vi "Frame Editor.vi"(8 "error in":errorcluster, 11 "Input File":path) -> (0 "error out":errorcluster, 1 "Cancelled":bool, 2 "Output Map":T3 {"value"."Type of Frame" items=["Raw Frame", "UDP/IP Tx Gen", "Tx UDP"]; "value"."Data" format="%.0x"}, 3 "Currently Loaded file":path)   [LabVIEW 2020, in "FrameEditor.lvlib"]
doc: "This template is for the Queued Message Handler design pattern.\n\nThe Event Handling Loop generates messages based on user interface actions.\n\nThe Message Handling Loop processes messages generated by the Event Handling Loop, or by other messages. The messages are string values, so new messages can be added easily to the Message Cases case structure in the Message Handling Loop. Each message cluster can also provide an optional value for Message Data, which is a variant that can be converted to whatever message-specific data is required."
uses:
  FrameEditor.lvlib
  controls/Type of Payload.ctl
  controls/Payload Map.ctl
  controls/Payload Record Type.ctl
  controls/UI Data.ctl
  <instrlib>/AIM GmbH/_AIM 664/helpers/EthFrameManagement/controls/arinc664_mac_src_info.ctl
  <instrlib>/AIM GmbH/_AIM 664/helpers/EthFrameManagement/controls/arinc664_ip_src_info.ctl
  support/Message Queue/Enqueue Message (Single).vi
  <instrlib>/AIM GmbH/_AIM 664/helpers/EthFrameManagement/Create Payload (Constant).vi
  <instrlib>/AIM GmbH/_AIM 664/helpers/EthFrameManagement/Create Payload (Increment).vi
  <instrlib>/AIM GmbH/_AIM 664/helpers/EthFrameManagement/Create Payload (Random).vi
  <vilib>/Utility/error.llb/Error Cluster From Error Code.vi
  <vilib>/ErrorRing/Error Ring.xnode
  support/Message Queue/Message Queue.lvlib
  support/User Event - Stop/User Event - Stop.lvlib
  <instrlib>/AIM GmbH/_AIM 664/AIM664LV.lvlib
  <instrlib>/AIM GmbH/_AIM 664/helpers/EthFrameManagement/EthFrameManagement.lvlib
panel:
  in  "Payloads":string(tree)
  in  "Header Information":T1={"Inter Frame Gap"=0, "Packet Group Wait Time"=10000, "Payload Buffer Mode"=0, "Payload Generation Mode"=0, "Preamble Count"=7, "Skew"=0, "Net Select"=4, "Frame Start Mode"=1, "Physical Error Injection"=0, "Sequence Number Init"=65535, "Sequence Number Offset"=65535} {"Net Select" items=["FDX_TX_FRAME_DLY_A"=0, "FDX_TX_FRAME_DLY_B"=1, "FDX_TX_FRAME_BOTH "=3, "FDX_TX_FRAME_ONLY_A"=4, "FDX_TX_FRAME_ONLY_B "=5]; "Frame Start Mode" items=["FDX_TX_FRAME_START_IFG", "FDX_TX_FRAME_START_PGWT", "FDX_TX_FRAME_START_TRG"]; "Physical Error Injection" items=["FDX_TX_FRAME_ERR_OFF"=0, "FDX_TX_FRAME_ERR_CRC"=1, "FDX_TX_FRAME_ERR_ALI"=2, "FDX_TX_FRAME_ERR_PRE"=4, "FDX_TX_FRAME_ERR_PHY"=8]; "Sequence Number Init" items=["FDX_TX_FRAME_SEQ_INIT_AUTO"=65535]; "Sequence Number Offset" items=["FDX_TX_FRAME_SEQ_OFFS_AUTO "=65535]; "Payload Generation Mode" items=["FDX_TX_FRAME_PGM_USER"=0, "FDX_TX_FRAME_PGM_IP_PART"=1, "FDX_TX_FRAME_PGM_IP_FULL"=2, "FDX_TX_FRAME_PGM_IP_PART_TT"=10, "FDX_TX_FRAME_PGM_IP_FULL_TT"=20]; "Payload Buffer Mode" items=["FDX_TX_FRAME_PBM_STD", "FDX_TX_FRAME_PBM_MAC", "FDX_TX_FRAME_PBM_UDP"]}
  in  "Type of Frame":T2=1 items=["Raw Frame", "UDP/IP Tx Gen", "Tx UDP"]
  out "option":u32
  in  "Payload ID":string
  in  "Tab Control":enum32{"Raw ", "Page 1", "Page 2"}(tab)
  out "Frame Size":u32=17
  in  "Headers":u8[](array[numeric])=[0, 0, 0, 0, 0, 0, 0, 0, 0, 0, 0, 0, 0, 0, 0, 0, 0] format="%02x"
  in  "UDP Source Port":u16=1
  in  "UDP Destination Port":u16=1
  in  "VL Id":u16=60
  in  "Domain ID":u8=1
  in  "Side ID":u8=1
  in  "Location ID":u8=1
  in  "Interface ID":u8=1
  in  "Partition ID":u8=1
  out "Source IP":string
  out "Destination MAC":string
  out "Source MAC":string
  out "Destination IP":string
  out "Frame Data":string[][](table)
  in  "Increment":u8=1 format="%.0x"
  in  "Start":u8=65 format="%02x"
  in  "Fill Value":u8=10 format="%02x"
  in  "Random Payload":bool
  in  "Increment Payload":bool
  in  "Fill Payload":bool
  in  "Bit Length":u16(ring) items=["Byte (8 bits)", "Word (16 bits)", "Long (32 bits)", "Quad (64 bits)"]
  in  "Clear Payload":bool
  in  "Payload Size":u32=17
  in  "Payload":u8[](array[numeric])=[0, 0, 0, 0, 0, 0, 0, 0, 0, 0, 0, 0, 0, 0, 0, 0, 0] format="%02x"
  in  "Cancel":bool
  in  "Load":bool
  in  "Save":bool
  in  "Remove":bool
  in  "Add / Update":bool
  in  "Exit":bool
  out "Display Message":string
  # "0-13 index: MAC Header\n14-34 index: IP Header\n35-43 index: UDP Header"
  # "Auto-generate Payload"
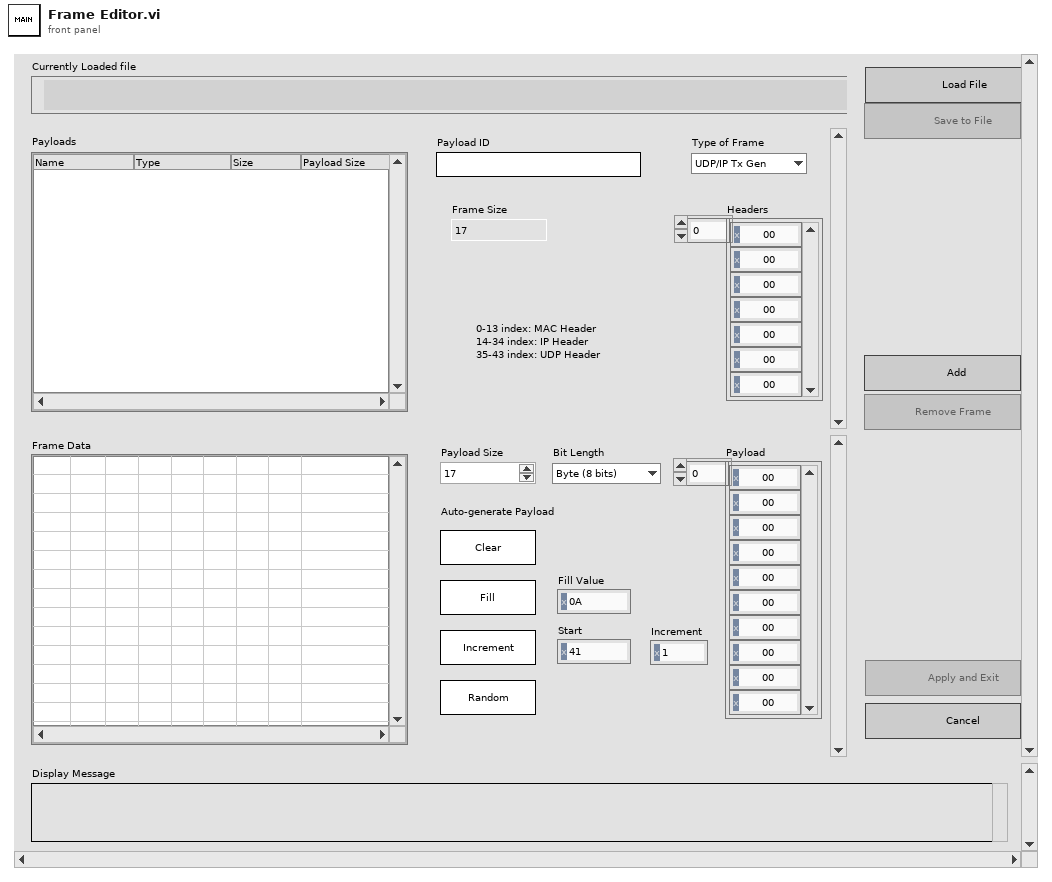
[diagram p1: front panel]
types:
  T1 = cluster{"Inter Frame Gap":u32, "Packet Group Wait Time":u32, "Payload Buffer Mode":u8, "Payload Generation Mode":u8, "Preamble Count":u8, "Skew":u32, "Net Select":u8, "Frame Start Mode":u8, "Physical Error Injection":u32, "Sequence Number Init":u16, "Sequence Number Offset":u16}
  T2 = typedef "Type of Payload.ctl" = u16
  T3 = typedef "Payload Map.ctl" = map{string, T4}
  T4 = typedef "Payload Record Type.ctl" = cluster{"Data":u8[], "Type of Frame":T2}
  T5 = typedef "UI Data.ctl" = cluster{"changesPending":bool, "String <Replace Me>":string, "Numeric <Replace Me>":dbl, "Add":refnum<vi>, "Remove":refnum<vi>, "Data Display Ref":refnum<vi>, "Exit Button Ref":refnum<vi>, "Load":refnum<vi>, "Save":refnum<vi>, "Payload ID":refnum<vi>, "Type of Frame":refnum<vi>}
  T6 = typedef "FrameEditor.lvlib/Message Queue.lvlib/All Message Queues.ctl" = cluster{"UI":refnum<queue>}
  T7 = cluster{"Left Cell String":string, "Child Text":string[], "Child Tag":string, "Item Indent":i32, "Child Only?":bool, "Glyph Index":i32}[]
  T8 = enum8{"Enabled", "Disabled", "Disabled and Grayed Out"}
  T9 = enum16{"open", "replace", "create", "open or create", "replace or create", "replace or create with confirmation"}
  T10 = typedef "EthFrameManagement.lvlib/arinc664_ip_src_info.ctl" = cluster{"domainID":u8, "sideID":u8, "locationID":u8, "partitionID":u8}
  T11 = typedef "EthFrameManagement.lvlib/arinc664_mac_src_info.ctl" = cluster{"domainID":u8, "sideID":u8, "locationID":u8, "interfaceID":u8}
  T12 = cluster{"Domain ID":u8, "Side ID":u8, "Location ID":u8, "Interface ID":u8, "Partition ID":u8}
  T13 = typedef "AIM664LV.lvlib/queue_data_full.ctl" = cluster{"domainID":u8, "sideID":u8, "locationID":u8, "interfaceID":u8, "partitionID":u8}
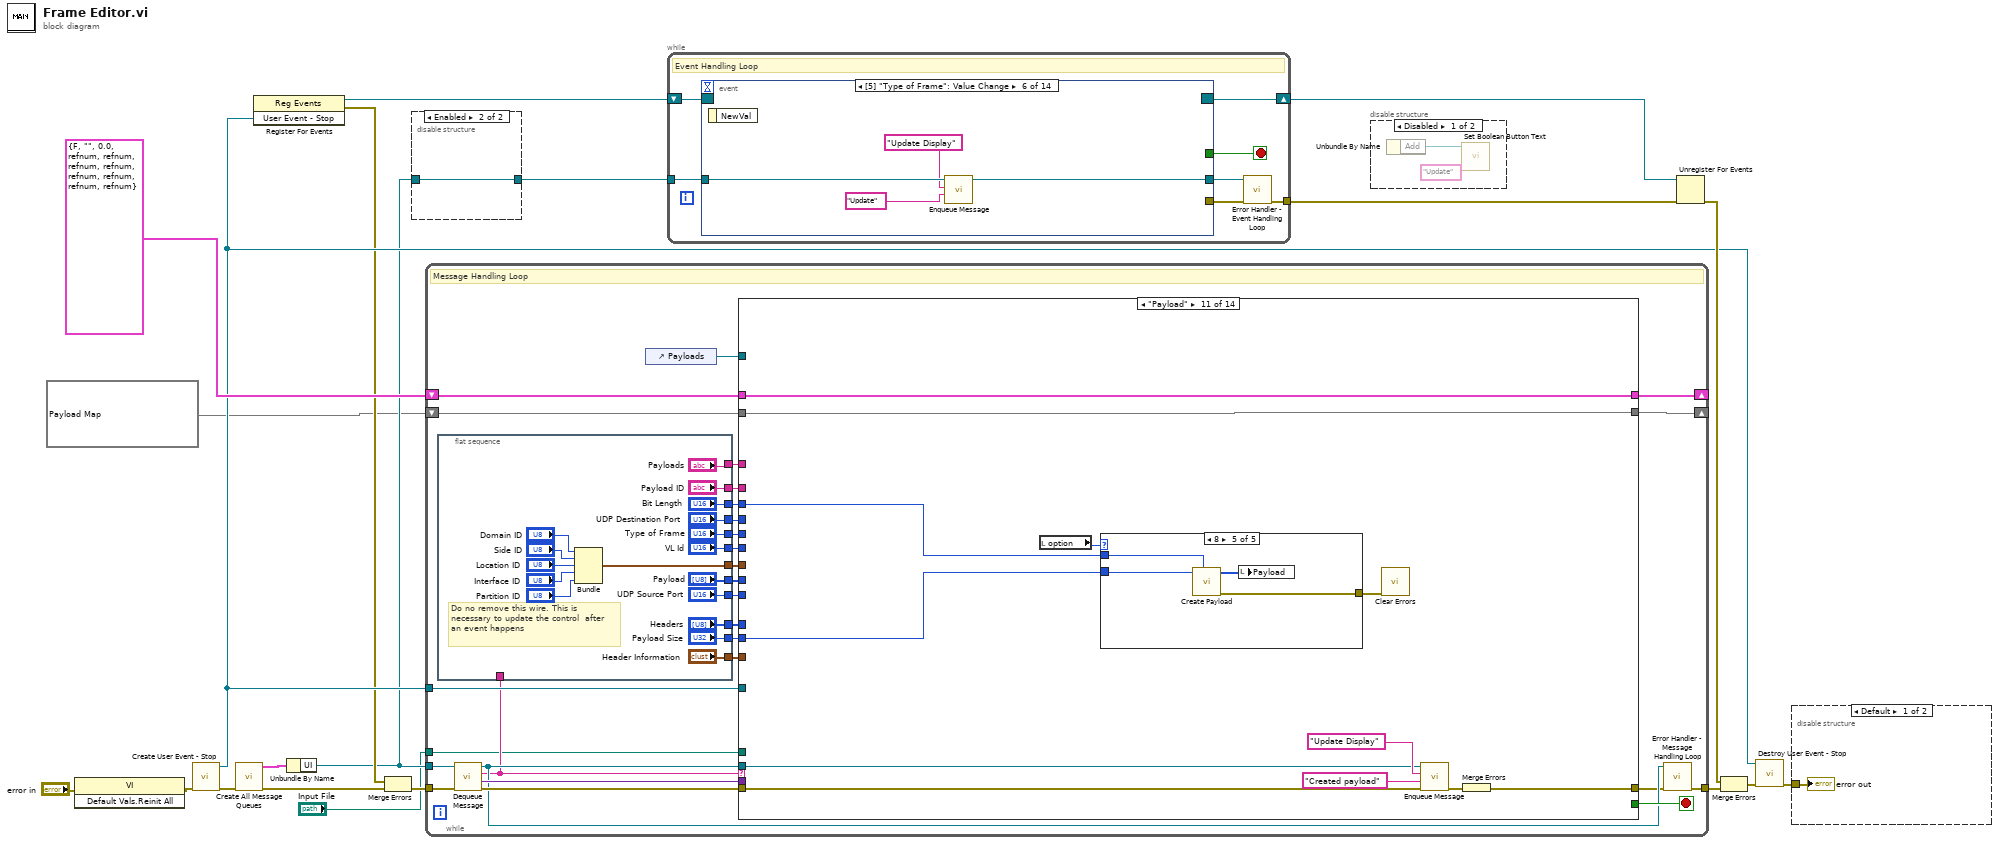
[diagram p0: block diagram]
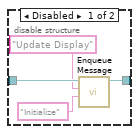
[diagram p3: hidden frame]
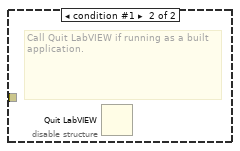
[diagram p4: hidden frame]
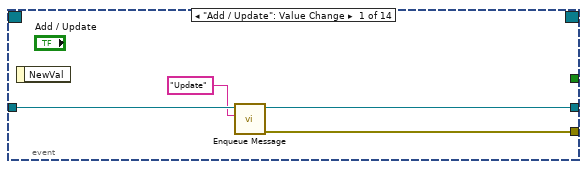
[diagram p5: hidden frame]
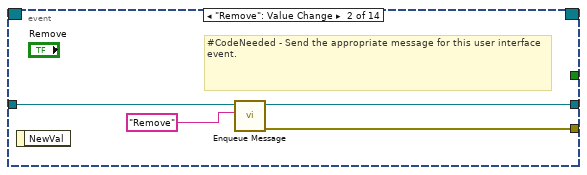
[diagram p6: hidden frame]
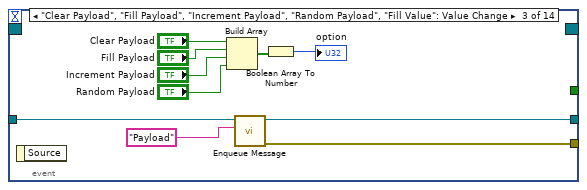
[diagram p7: hidden frame]
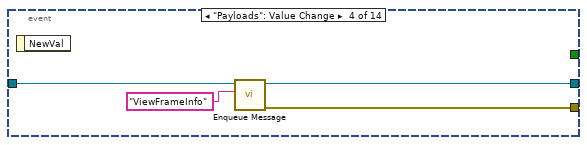
[diagram p8: hidden frame]
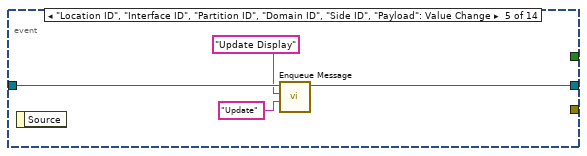
[diagram p9: hidden frame]
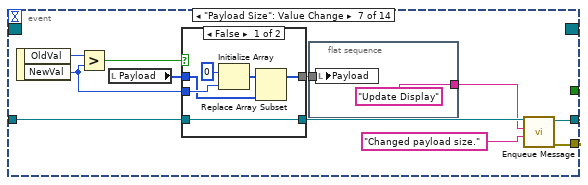
[diagram p10: hidden frame]
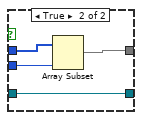
[diagram p11: hidden frame]
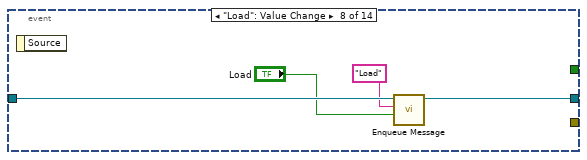
[diagram p12: hidden frame]
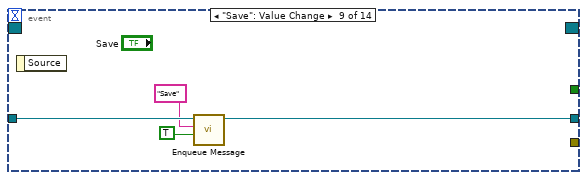
[diagram p13: hidden frame]
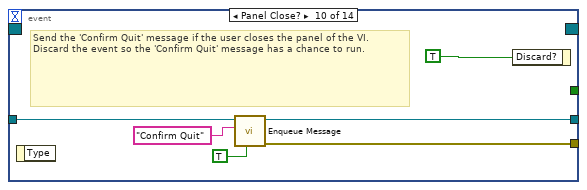
[diagram p14: hidden frame]
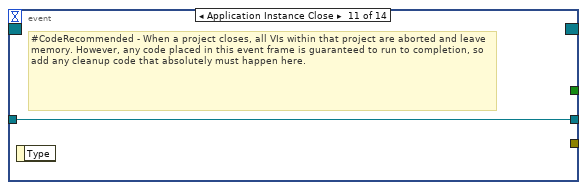
[diagram p15: hidden frame]
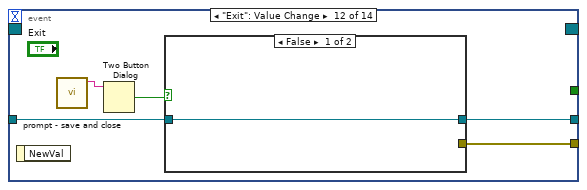
[diagram p16: hidden frame]
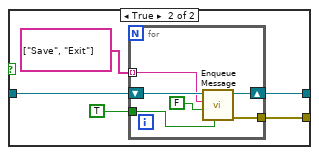
[diagram p17: hidden frame]
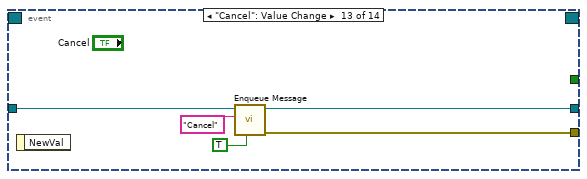
[diagram p18: hidden frame]
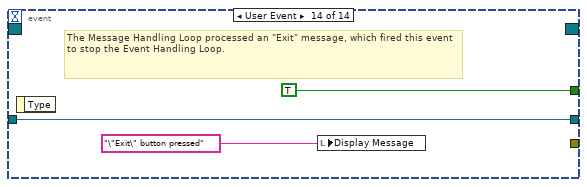
[diagram p19: hidden frame]
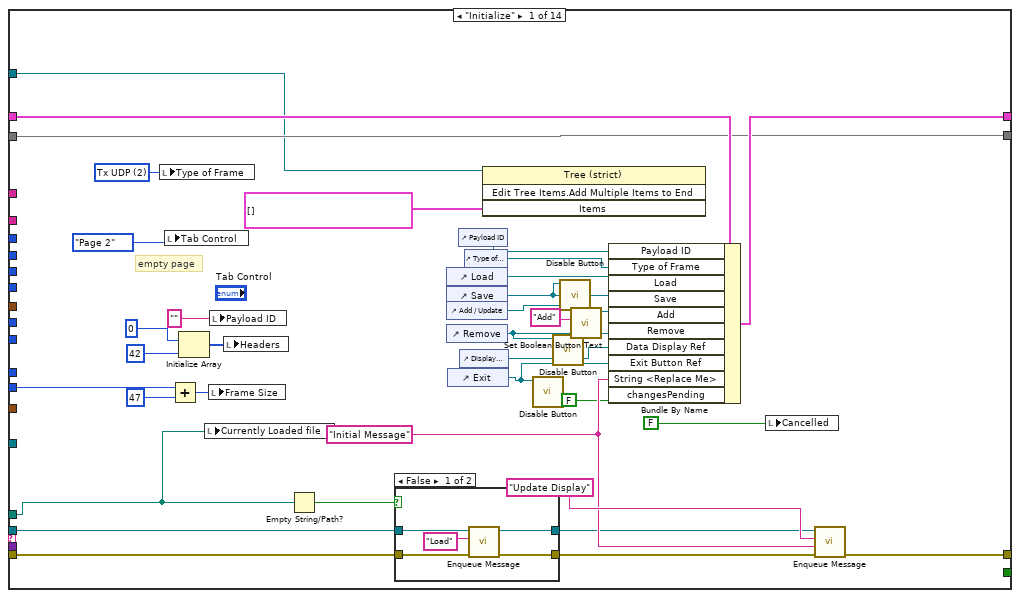
[diagram p20: hidden frame]
diagram:
  n1 = invoke class="VI" method="Default Vals.Reinit All"(error in="error in") -> (error out=w4:errorcluster)  [unwired: 2 in, 2 out]
  n2 = call "Create User Event - Stop.vi"("error in (no error)"=w4) -> ("error out"=w17:errorcluster, "User Event - Stop"=w9:refnum<user-event>)  [unwired: 9 in]
  n3 = call "Create All Message Queues.vi"("error in (no error)"=w17) -> ("error out"=w20:errorcluster, "Message Queues out"=w19:T6)  [unwired: 9 in]
  n4 = register-events(w9) -> (reference out=w10:refnum<event-registration>, error out=w7:errorcluster)  [unwired: 2 in]
  n5 = Unbundle By Name(w19) -> ("UI"=w6:refnum<queue>)
  n6 = Merge Errors(w7, w20) -> (w8:errorcluster)
  n7 = disable-structure shown="Enabled" {
    disable-tunnel: w6 -> [w24 w25]
    disable-tunnel: [w23 w25] -> w5
    frame Disabled {
      n8 = call-poly "Enqueue Message.vi"("Message Data"="Initialize" ("Message"), "Message"="Update Display", "Message Queue"=w24) -> ("dup Message Queue"=w23:refnum<queue>)  [unwired: 7 in, 1 out]
    }
    frame Enabled {
    }
  }
  n9 = while {
    tunnel: w6 -> [w46]
    shift-right: [w52] -> _
    shift-left: T5 {"changesPending"=FALSE, "String <Replace Me>"="", "Numeric <Replace Me>"=0.0, "Add"=refnum, "Remove"=refnum, "Data Display Ref"=refnum, "Exit Button Ref"=refnum, "Load"=refnum, "Save"=refnum, "Payload ID"=refnum, "Type of Frame"=refnum} ("Data Cluster") -> [w53]
    tunnel: w9 -> [w50]
    tunnel: w8 -> [w49]
    tunnel: [w44] -> w18
    shift-right: [w33] -> _
    shift-left: T3 {} -> [w35]
    tunnel: "Input File" -> [w26]
    stop <- w51 stop-if-true
    # "Message Handling Loop"
    n10 = flat-sequence {
      tunnel: ["Payload Size"] -> w42
      tunnel: [w69] -> w41
      tunnel: ["VL Id"] -> w40
      tunnel: ["UDP Source Port"] -> w39
      tunnel: ["UDP Destination Port"] -> w38
      tunnel: ["Payload"] -> w37
      tunnel: ["Header Information"] -> w36
      tunnel: ["Payload ID"] -> w34
      tunnel: ["Payloads"] -> w32
      tunnel: ["Bit Length"] -> w31
      tunnel: w30 -> [_]
      tunnel: ["Type of Frame"] -> w28
      tunnel: ["Headers"] -> w27
      frame #0 {
        # "Do no remove this wire. This is necessary to update the control  after an event happens"
        n11 = Bundle("Domain ID"="Domain ID", "Side ID"="Side ID", "Location ID"="Location ID", "Interface ID"="Interface ID", "Partition ID"="Partition ID") -> (w69:T12)  [unwired: 1 in]
      }
    }
    n12 = call "Dequeue Message.vi"("error in (no error)"=w49, "Message Queue"=w46) -> ("error out"=w48:errorcluster, "Message Data"=w47:variant, "Message"=w30:string, "dup Message Queue"=w45:refnum<queue>)  [unwired: 6 in]
    n13 = control-ref of="Payloads"() -> (w29:refnum<vi>)
    n14 = case "Message Cases" shown="\"Payload\"" w30 {
      selector: w30 -> [_ _ _ _ _ _ _ _ _ _ _ _ _ w515]
      tunnel: w45 -> [w88 w137 w209 w223 w260 w329 _ _ w448 _ w459 w500 w513 _]
      tunnel: w48 -> [w86 w139 w211 w225 w251 w326 w422 w444 w452 w456 w462 w493 w506 _]
      tunnel: [w105 w140 w212 w226 w261 w331 w423 w439 w450 w454 w467 w496 w509 w516] -> w43
      tunnel: w53 -> [w104 w116 w196 w215 w257 w332 w383 w443 w451 w455 w468 w499 w512 w517]
      tunnel: [w103 w115 w195 w215 w255 w332 w383 w443 w451 w455 w468 w499 w512 w517] -> w52
      tunnel: [_ _ _ _ _ _ _ _ _ _ _ TRUE TRUE _] -> w51
      tunnel: w47 -> [_ _ _ _ w254 w321 w421 w442 _ _ _ w490 w503 _]
      tunnel: w50 -> [_ _ _ _ _ _ _ _ _ _ _ w495 w508 _]
      tunnel: w42 -> [w91 w124 _ _ _ _ _ _ _ _ w465 _ _ _]
      tunnel: w41 -> [_ w134 _ _ _ _ w406 _ _ _ _ _ _ _]
      tunnel: w40 -> [_ w135 _ _ _ _ w407 _ _ _ _ _ _ _]
      tunnel: w39 -> [_ w131 _ _ _ _ _ _ _ _ _ _ _ _]
      tunnel: w38 -> [_ w133 _ _ _ _ _ _ _ _ _ _ _ _]
      tunnel: w37 -> [_ w132 _ _ _ _ _ _ _ _ _ _ _ _]
      tunnel: w36 -> [_ _ _ _ _ _ _ _ _ _ _ _ _ _]
      tunnel: w35 -> [w98 w123 w203 w221 w256 w324 w393 w438 w445 w453 w466 w489 w502 w514]
      tunnel: w34 -> [_ w114 _ _ _ _ w392 _ _ _ _ _ _ _]
      tunnel: [w98 w127 w206 w221 w256 w325 w393 w438 w445 w453 w466 w489 w502 w514] -> w33
      tunnel: w32 -> [_ w113 w202 w216 _ _ w389 _ _ _ _ _ _ _]
      tunnel: w29 -> [w96 w117 w207 w222 _ w327 w395 _ _ _ _ _ _ _]
      tunnel: w31 -> [_ _ _ _ _ _ w417 _ _ _ w464 _ _ _]
      tunnel: w28 -> [_ w125 _ _ _ _ w382 _ _ _ _ _ _ _]
      tunnel: w27 -> [_ w126 _ _ _ _ _ _ _ _ _ _ _ _]
      tunnel: w26 -> [w83 _ _ _ _ _ _ _ _ _ _ _ _ _]
      frame "Initialize" {
        w71 = T2 2 items=["Raw Frame", "UDP/IP Tx Gen", "Tx UDP"] ("Type of Frame")
        w100 = "Initial Message" ("Initial Message")
        # "empty page"
        # "Initialize - All initialization work should take place in this message, since other loops can potentially enqueue messages that execute immediately after this one."
        n15 = local write "Type of Frame"(w71) -> ()
        n16 = local write "Tab Control"(enum32{"Raw ", "Page 1", "Page 2"}."Page 2" ("Tab Control")) -> ()
        n17 = Add(x=w91, y=u32 47) -> (x+y=w89:u32)
        n18 = Initialize Array(u32 0 ("element"), 42 ("dimension size")) -> (w94:u32[])
        n19 = local write "Currently Loaded file"(w83) -> ()
        n20 = local write "Frame Size"(w89) -> ()
        n21 = local write "Payload ID"("" ("Payload ID")) -> ()
        n22 = local write "Headers"(w94) -> ()
        n23 = Empty String/Path?(string/path=w83) -> (empty?=w84:bool)
        n24 = case shown="False" w84 {
          tunnel: w88 -> [w109 w112]
          tunnel: [w108 w112] -> w87
          tunnel: w86 -> [w107 w111]
          tunnel: [w106 w111] -> w85
          frame False {
            n25 = call-poly "Enqueue Message.vi"("error in (no error)"=w107, "Message"="Load", "Message Queue"=w109) -> ("error out"=w106:errorcluster, "dup Message Queue"=w108:refnum<queue>)  [unwired: 7 in]
          }
          frame True {
          }
        }
        n26 = control-ref of="Load"() -> (w99:refnum<vi>)
        n27 = control-ref of="Save"() -> (w72:refnum<vi>)
        n28 = control-ref of="Add / Update"() -> (w81:refnum<vi>)
        n29 = control-ref of="Remove"() -> (w77:refnum<vi>)
        n30 = control-ref of="Exit"() -> (w73:refnum<vi>)
        n31 = control-ref of="Payload ID"() -> (w76:refnum<vi>)
        n32 = control-ref of="Display Message"() -> (w102:refnum<vi>)
        n33 = control-ref of="Type of Frame"() -> (w75:refnum<vi>)
        n34 = invoke on="Invoke Node" class="Tree (strict)" method="Edit Tree Items.Add Multiple Items to End"(reference=w96, "Items"=T7 []) -> ()  [unwired: 2 in, 4 out]
        n35 = call "Disable Button.vi"("ctrl ref in"=w73) -> ()  [unwired: 11 in]
        n36 = call "Disable Button.vi"("ctrl ref in"=w77) -> ()  [unwired: 11 in]
        n37 = call "Disable Button.vi"("ctrl ref in"=w72) -> ()  [unwired: 11 in]
        n38 = call "Set Boolean Button Text.vi"("text"="Add", "boolean ref in"=w81) -> ("bool ref out"=w80:refnum<vi>)  [unwired: 9 in]
        n39 = Bundle By Name(cluster=w104, "Payload ID"=w76, "Type of Frame"=w75, "Load"=w99, "Save"=w72, "Add"=w80, "Remove"=w77, "Data Display Ref"=w102, "Exit Button Ref"=w73, "String <Replace Me>"=w100, "changesPending"=FALSE) -> (w103:T5)
        n40 = local write "Cancelled"(FALSE ("Cancel")) -> ()
        n41 = call-poly "Enqueue Message.vi"("error in (no error)"=w85, "Message Data"=w100, "Message"="Update Display", "Message Queue"=w87) -> ("error out"=w105:errorcluster)  [unwired: 6 in, 1 out]
      }
      frame "Update" {
        # "Something - Replace this message with functionality for your own application."
        n42 = case shown="1" w125 {
          tunnel: w135 -> [_ w155 _]
          tunnel: w134 -> [_ w154 _]
          tunnel: w133 -> [_ w153 _]
          tunnel: w132 -> [w146 w152 w156]
          tunnel: w131 -> [_ w151 _]
          tunnel: [w145 w150 w156] -> w130
          tunnel: w126 -> [w141 _ _]
          tunnel: w124 -> [w144 _ _]
          frame 0, Default {
            n43 = Add(x=w144, y=u32 47) -> (x+y=w142:u32)
            "Frame Size" <- w142
            n44 = Initialize Array(u32 0 ("element"), w142) -> (w148:u32[])
            n45 = Replace Array Subset(array=w148, new element=w141) -> (w147:u32[])  [unwired: 1 in]
            n46 = call <instrlib>:"WritePayload(UDP).vi"("Payload"=w146, "Ethernet Frame In"=w147) -> ("Ethernet Frame Out"=w145:u8[])  [unwired: 8 in, 1 out]
          }
          frame 1 {
            n47 = call <instrlib>:"FdxCreateTxQueueDataFrame.vi"("UDPsrcPort"=w151, "UDPdstPort"=w153, "Payload"=w152, "afdx configuration"=w154, "VL Id"=w155) -> ("Frame"=w150:u8[])  [unwired: 4 in, 2 out]
          }
          frame 2 {
          }
        }
        n48 = Look In Map(map=w123, key=w114) -> (key not found?=w120:bool)  [unwired: 1 in, 1 out]
        n49 = Empty String/Path?(string/path=w113) -> (empty?=w119:bool)
        n50 = And(x=w120, y=w119) -> (x .and. y?=w121:bool)
        n51 = Empty String/Path?(string/path=w114) -> (empty?=w129:bool)
        n52 = Bundle By Name(cluster=T4 {"Data"=[], "Type of Frame"=0} ("value"), "Type of Frame"=w125, "Data"=w130) -> (w128:T4)
        n53 = case shown="False" w129 {
          tunnel: w114 -> [w166 _]
          tunnel: w123 -> [w167 w194]
          tunnel: [w160 w194] -> w127
          tunnel: w128 -> [w165 _]
          tunnel: [w164 w193] -> w122
          tunnel: w121 -> [w163 _]
          tunnel: w119 -> [w162 _]
          tunnel: w117 -> [w161 _]
          tunnel: w116 -> [w159 w192]
          tunnel: [w158 w192] -> w115
          tunnel: w113 -> [w157 _]
          frame False {
            n54 = case shown="False" w163 {
              tunnel: w167 -> [w171 w191]
              tunnel: w166 -> [w170 w190]
              tunnel: [w172 w189] -> w160
              tunnel: w165 -> [w169 w188]
              tunnel: [w173 w184] -> w164
              tunnel: w162 -> [w174 _]
              tunnel: w157 -> [w168 _]
              frame False {
                n55 = case shown="False" w174 {
                  tunnel: [w178 w183] -> w173
                  tunnel: [w181 w182] -> w172
                  tunnel: w171 -> [w177 w182]
                  tunnel: w170 -> [w180 _]
                  tunnel: w169 -> [w179 _]
                  tunnel: w168 -> [w176 _]
                  frame False {
                    n56 = Remove From Map(10:w176, 11:w177) -> (3:w175:T3)  [unwired: 2 out]
                    n57 = call "prompt - frame updated.vi"() -> ("message"=w178:string)  [unwired: 11 in]
                    n58 = Insert Into Map(map in=w175, key=w180, value=w179) -> (map out=w181:T3)  [unwired: 2 out]
                  }
                  frame True {
                    n59 = call "prompt - frame exists.vi"() -> ("message"=w183:string)  [unwired: 11 in]
                  }
                }
              }
              frame True {
                # "add new"
                n60 = call "prompt - frame updated.vi"() -> ("message"=w186:string)  [unwired: 11 in]
                n61 = call "prompt - frame added.vi"() -> ("message"=w185:string)  [unwired: 11 in]
                n62 = Insert Into Map(map in=w191, key=w190, value=w188) -> (map out=w189:T3, key already included?=w187:bool)  [unwired: 1 out]
                n63 = Select(t=w186, s=w187, f=w185) -> (s? t:f=w184:string)
              }
            }
            n64 = call "Set Pending Changes.vi"("Data Cluster in"=w159) -> ("Data Cluster out"=w158:T5)  [unwired: 10 in]
            n65 = call "Update Tree Control.vi"("frame map"=w160, "Tree 2"=w161) -> ()  [unwired: 10 in]
          }
          frame True {
            n66 = call "prompt - payload not found.vi"() -> ("message"=w193:string)  [unwired: 11 in]
            n67 = One Button Dialog(message=w193) -> ()  [unwired: 1 in, 1 out]
          }
        }
        n68 = call-poly "Enqueue Message.vi"("error in (no error)"=w139, "Message Data"=w122, "Message"="Update Display", "Message Queue"=w137) -> ("error out"=w138:errorcluster)  [unwired: 6 in, 1 out]
        n69 = Merge Errors(w138) -> (w140:errorcluster)
      }
      frame "Remove" {
        # "Something Else - Replace this message with functionality for your own application."
        n70 = invoke on="Payload ID" class="Str" method="Reinit To Default"() -> ()  [unwired: 3 in, 3 out]
        n71 = invoke on="UDP Destination Port" class="DigNum (strict)" method="Reinit To Default"() -> ()  [unwired: 3 in, 3 out]
        n72 = invoke on="VL Id" class="DigNum (strict)" method="Reinit To Default"() -> ()  [unwired: 3 in, 3 out]
        n73 = local write "Payloads"("" ("Payloads")) -> ()
        n74 = Equal?(x=w202, y="") -> (x = y?=w205:bool)
        n75 = case shown="True" w205 {
          tunnel: ["Frame removed." ("format string") "Frame was not selected, so no Frames were removed." ("format string")] -> w204
          frame False {
          }
          frame True {
          }
        }
        n76 = invoke on="UDP Source Port" class="DigNum (strict)" method="Reinit To Default"() -> ()  [unwired: 3 in, 3 out]
        n77 = invoke on="Payload" class="Arr (strict)" method="Reinit To Default"() -> ()  [unwired: 3 in, 3 out]
        n78 = invoke on="Payload Size" class="DigNum (strict)" method="Reinit To Default"() -> ()  [unwired: 3 in, 3 out]
        n79 = invoke on="Header Information" class="Clust (strict)" method="Reinit To Default"() -> ()  [unwired: 3 in, 3 out]
        n80 = Remove From Map(10:w202, 11:w203) -> (3:w206:T3)  [unwired: 2 out]
        n81 = call "Update Tree Control.vi"("frame map"=w206, "Tree 2"=w207) -> ()  [unwired: 10 in]
        n82 = Unbundle By Name(w196) -> ("Remove"=w200:refnum<vi>, "Add"=w199:refnum<vi>)
        n83 = call "Set Pending Changes.vi"("Data Cluster in"=w196) -> ("Data Cluster out"=w195:T5)  [unwired: 10 in]
        n84 = call-poly "Enqueue Message.vi"("error in (no error)"=w211, "Message Data"=w204, "Message"="Update Display", "Message Queue"=w209) -> ("error out"=w210:errorcluster)  [unwired: 6 in, 1 out]
        n85 = call "Disable Button.vi"("ctrl ref in"=w200) -> ()  [unwired: 11 in]
        n86 = call "Set Boolean Button Text.vi"("text"="Add", "boolean ref in"=w199) -> ()  [unwired: 9 in, 1 out]
        n87 = Merge Errors(w210) -> (w212:errorcluster)
      }
      frame "ViewFrameInfo" {
        # "Something Else - Replace this message with functionality for your own application."
        n88 = Look In Map(map=w221, key=w216) -> (key not found?=w220:bool, value=w219:T4)  [unwired: 1 in]
        n89 = call "Update Tree Control.vi"("frame map"=w221, "Tree 2"=w222) -> ()  [unwired: 10 in]
        n90 = case shown="False" w220 {
          tunnel: w219 -> [w246 _]
          tunnel: [w244 "Frame not found"] -> w217
          tunnel: w216 -> [w238 _]
          tunnel: w215 -> [w230 w247]
          frame False {
            n91 = Unbundle By Name(w246) -> ("Data"=w242:u8[], "Type of Frame"=w227:T2)
            n92 = Unbundle By Name(w230) -> ("Remove"=w229:refnum<vi>)
            n93 = local write "Payload ID"(w238) -> ()
            n94 = call "Disable Button.vi"("Disabled"=T8."Enabled", "ctrl ref in"=w229) -> ()  [unwired: 10 in]
            n95 = call "Parse Raw Payload Frame.vi"("Data"=w242) -> ("UDPsrcPort"=w239:u16, "UDPdstPort"=w240:u16, "VL Id"=w241:u16, "Payload"=w232:u8[], "Frame Configuration"=w243:T13)  [unwired: 6 in]
            n96 = Format Into String(format string="Frame %s displayed", w238) -> (resulting string=w244:string)  [unwired: 2 in, 1 out]
            n97 = Unbundle(w243) -> ("domainID"=w237:u8, "sideID"=w233:u8, "locationID"=w236:u8, "interfaceID"=w234:u8, "partitionID"=w235:u8)
            n98 = Array Size(array=w232) -> (size(s)=w231:i32)
            n99 = local write "UDP Destination Port"(w240) -> ()
            n100 = local write "UDP Source Port"(w239) -> ()
            n101 = local write "Type of Frame"(w227) -> ()
            n102 = local write "Payload Size"(w231) -> ()
            n103 = local write "Tab Control"(w227) -> ()
            n104 = local write "Location ID"(w236) -> ()
            n105 = local write "Interface ID"(w234) -> ()
            n106 = local write "Partition ID"(w235) -> ()
            n107 = local write "Domain ID"(w237) -> ()
            n108 = local write "Payload"(w232) -> ()
            n109 = local write "Side ID"(w233) -> ()
            n110 = local write "VL Id"(w241) -> ()
          }
          frame True {
            n111 = Unbundle By Name(w247) -> ("Remove"=w248:refnum<vi>)
            n112 = call "Disable Button.vi"("ctrl ref in"=w248) -> ()  [unwired: 11 in]
          }
        }
        n113 = call-poly "Enqueue Message.vi"("error in (no error)"=w225, "Message Data"=w217, "Message"="Update Display", "Message Queue"=w223) -> ("error out"=w224:errorcluster)  [unwired: 6 in, 1 out]
        n114 = Merge Errors(w224) -> (w226:errorcluster)
      }
      frame "Save" {
        # "Something Else - Replace this message with functionality for your own application."
        n115 = Variant To Data(error in=w251, type=FALSE, Variant=w254) -> (data=w252:bool, error out=w250:errorcluster)
        n116 = case shown="True" w252 {
          tunnel: [TRUE ("T button?") w266] -> w259
          tunnel: [w263 w265] -> w258
          frame False {
            n117 = local read "Currently Loaded file"() -> (w263:path)
          }
          frame True {
            n118 = local read "Currently Loaded file"() -> (w265:path)
            n119 = call "prompt - file save.vi"("Path"=w265) -> ("message"=w264:string)  [unwired: 10 in]
            n120 = Two Button Dialog(message=w264) -> (T button?=w266:bool)  [unwired: 2 in]
          }
        }
        n121 = case shown="True" w259 {
          tunnel: [w268 w278] -> w261
          tunnel: w260 -> [_ w277]
          tunnel: w250 -> [w268 w276]
          tunnel: w256 -> [_ w275]
          tunnel: w258 -> [_ w274]
          tunnel: w257 -> [w267 w271]
          tunnel: [w267 w270] -> w255
          frame False {
          }
          frame True {
            n122 = call "File Dialog"("start path"=w274, "pattern (all files)"="*.bin") -> ("selected path"=w273:path, "cancelled"=w272:bool)  [unwired: 10 in, 2 out]
            n123 = case shown="False" w272 {
              tunnel: [w296 w312] -> w278
              tunnel: w277 -> [w294 _]
              tunnel: w276 -> [w292 w312]
              tunnel: w275 -> [w291 _]
              tunnel: w273 -> [w281 _]
              tunnel: w271 -> [w279 w311]
              tunnel: [w280 w311] -> w270
              frame False {
                n124 = for {
                  tunnel: w291 -> [w310] mode=indexing
                  tunnel: [w307] -> w288 mode=indexing
                  n125 = Unbundle By Name(w310) -> ("key"=w309:string, "value"=w308:T4)
                  n126 = Bundle("key"=w309, "value"=w308) -> (w307:cluster{"key":string, "value":T4})  [unwired: 1 in]
                }
                n127 = Open/Create/Replace File(file path (use dialog)=w281, error in=w292, operation (0:open)=T9."replace or create") -> (refnum out=w290:refnum<file>, error out=w283:errorcluster)  [unwired: 3 in, 1 out]
                n128 = case shown="No Error" w283 {
                  selector: w283 -> [w297 w305]
                  tunnel: w290 -> [w303 _]
                  tunnel: [w300 w304] -> w289
                  tunnel: w288 -> [w299 _]
                  tunnel: [w298 _] -> w285
                  tunnel: [w297 w304] -> w282
                  frame No Error {
                    n129 = Write to Binary File(file (use dialog)=w303, data=w299, error in=w297) -> (refnum out=w301:refnum<file>, error out=w302:errorcluster)  [unwired: 3 in, 1 out]
                    n130 = Close File(refnum=w301, error in=w302) -> (path=w298:path, error out=w300:errorcluster)
                  }
                  frame Error {
                    n131 = call <vilib>:"Clear Errors.vi"("error in (no error)"=w305, "specific error code to clear (0: all)"=43) -> ("error out"=w304:errorcluster)  [unwired: 4 in, 1 out]
                  }
                }
                "Currently Loaded file" <- w285
                n132 = Format Into String(format string="File %s Saved", w285) -> (resulting string=w287:string)  [unwired: 2 in, 1 out]
                n133 = call-poly "Enqueue Message.vi"("error in (no error)"=w282, "Message Data"=w287, "Message"="Update Display", "Message Queue"=w294) -> ("error out"=w295:errorcluster)  [unwired: 6 in, 1 out]
                n134 = call "Reset Pending Changes.vi"("Data Cluster in"=w279) -> ("Data Cluster out"=w280:T5)  [unwired: 10 in]
                n135 = Merge Errors(w289, w295) -> (w296:errorcluster)
              }
              frame True {
              }
            }
          }
        }
      }
      frame "Load" {
        # "Something - Replace this message with functionality for your own application."
        n136 = local read "Currently Loaded file"() -> (w316:path)
        n137 = Variant To Data(type=FALSE, Variant=w321) -> (data=w319:bool)  [unwired: 1 in, 1 out]
        n138 = Empty String/Path?(string/path=w316) -> (empty?=w323:bool)
        n139 = Or(x=w323, y=w319) -> (x .or. y?=w322:bool)
        n140 = case shown="True" w322 {
          tunnel: w326 -> [w338 w343]
          tunnel: [w335 w342] -> w313
          tunnel: [w336 w343] -> w315
          tunnel: w316 -> [w339 w342]
          tunnel: [T9."replace or create" ("operation (0:open)") T9."open" ("operation (0:open)")] -> _
          tunnel: [w333 FALSE ("cancelled")] -> w314
          frame True {
            n141 = call "File Dialog2"("start path"=w339, "error in"=w338, "pattern (all files)"="*.bin") -> ("selected path"=w335:path, "cancelled"=w333:bool, "error out"=w336:errorcluster)  [unwired: 9 in, 1 out]
          }
          frame False {
          }
        }
        n142 = case shown="False" w314 {
          tunnel: w327 -> [w356 _]
          tunnel: [w352 w381] -> w325
          tunnel: w324 -> [w351 w381]
          tunnel: [w348 w378] -> w318
          tunnel: [w357 "Load Cancelled." ("format string")] -> w317
          tunnel: w315 -> [w347 w379]
          tunnel: w313 -> [w344 _]
          frame False {
            n143 = Open/Create/Replace File(file path (use dialog)=w344, error in=w347) -> (refnum out=w345:refnum<file>, error out=w346:errorcluster)  [unwired: 4 in, 1 out]
            n144 = Read from Binary File(5:cluster{"FrameID":string, "value":T4}[] [], 8:w346, 11:w345) -> (0:w355:errorcluster, 2:w358:cluster{"FrameID":string, "value":T4}[], 3:w350:refnum<file>)  [unwired: 3 in, 1 out]
            n145 = case shown="No Error" w355 {
              selector: w355 -> [w363 w376]
              tunnel: w358 -> [w366 _]
              tunnel: [w360 w373] -> w352
              tunnel: [w364 w374] -> w357
              tunnel: [w363 w375] -> w349
              tunnel: w356 -> [w362 _]
              tunnel: T3 {} -> [w361 _]
              tunnel: w351 -> [_ w373]
              tunnel: w344 -> [w359 w372]
              frame No Error {
                n146 = for {
                  shift-right: [w370] -> w360
                  shift-left: w361 -> [w371]
                  tunnel: w366 -> [w369] mode=indexing
                  n147 = Unbundle By Name(w369) -> ("FrameID"=w368:string, "value"=w367:T4)
                  n148 = Insert Into Map(map in=w371, key=w368, value=w367) -> (map out=w370:T3)  [unwired: 2 out]
                }
                n149 = local write "Currently Loaded file"(w359) -> ()
                n150 = Format Into String(format string="File %s Loaded", w359) -> (resulting string=w364:string)  [unwired: 2 in, 1 out]
                n151 = call "Update Tree Control.vi"("frame map"=w360, "Tree 2"=w362) -> ()  [unwired: 10 in]
              }
              frame Error {
                # "Any error, we keep what we \nhad before."
                n152 = call <vilib>:"Simple Error Handler.vi"("error in (no error)"=w376) -> ("error out"=w375:errorcluster)  [unwired: 4 in, 4 out]
                n153 = Format Into String(format string="Error Loading %s", w372) -> (resulting string=w374:string)  [unwired: 2 in, 1 out]
              }
            }
            n154 = Close File(refnum=w350, error in=w349) -> (error out=w348:errorcluster)  [unwired: 1 out]
          }
          frame True {
            n155 = call <vilib>:"Clear Errors.vi"("error in (no error)"=w379) -> ("error out"=w378:errorcluster)  [unwired: 5 in, 1 out]
          }
        }
        n156 = call-poly "Enqueue Message.vi"("error in (no error)"=w326, "Message Data"=w317, "Message"="Update Display", "Message Queue"=w329) -> ("error out"=w330:errorcluster)  [unwired: 6 in, 1 out]
        n157 = Merge Errors(w318, w330) -> (w331:errorcluster)
      }
      frame "Update Display" {
        # "Update Display - Convert the message data to a string to display in the Data Display indicator."
        n158 = call "Update Tree Control.vi"("frame map"=w393, "Tree 2"=w395) -> ()  [unwired: 10 in]
        n159 = local write "Tab Control"(w382) -> ()
        n160 = Unbundle By Name(w383) -> ("Add"=w388:refnum<vi>)
        n161 = Empty String/Path?(string/path=w389) -> (empty?=w387:bool)
        n162 = Variant To Data(error in=w422, type="", Variant=w421) -> (data=→"Display Message":string, error out=w419:errorcluster)
        n163 = Look In Map(map=w393, key=w392) -> (key not found?=w390:bool, value=w391:T4)  [unwired: 1 in]
        n164 = case shown="False" w390 {
          tunnel: w417 -> [w430 _]
          tunnel: [w427 _] -> w394
          tunnel: w391 -> [w425 _]
          frame False {
            n165 = Unbundle By Name(w425) -> ("Data"=w424:u8[])
            n166 = Increment(x=w430) -> (x+1=w428:u16)
            n167 = Multiply(x=w428, y=u16 8) -> (x*y=w426:u16)
            n168 = call "Convert Non-visible Char to Visible Char.vi"("bytes per row"=w426, "data"=w424) -> ("data table"=w427:string[][])  [unwired: 7 in, 2 out]
          }
          frame True {
          }
        }
        "Frame Data" <- w394
        n169 = Select(t="Add", s=w387, f="Update") -> (s? t:f=w386:string)
        n170 = call "Set Boolean Button Text.vi"("text"=w386, "boolean ref in"=w388) -> ()  [unwired: 9 in, 1 out]
        n171 = Unbundle By Name(w406) -> ("Domain ID"=w411:u8, "Side ID"=w410:u8, "Location ID"=w409:u8, "Interface ID"=w414:u8, "Partition ID"=w408:u8)
        n172 = call <instrlib>:"Create ARINC-664 MAC (Dest).vi"("VL Id"=w407) -> ("MAC-src"=w401:u8[])  [unwired: 9 in, 1 out]
        n173 = call <instrlib>:"Create ARINC-664 IP (Dest).vi"("VL"=w407) -> ("ip string"=→"Destination IP":string)  [unwired: 8 in, 2 out]
        n174 = Bundle By Name(cluster=T11 {"domainID"=0, "sideID"=0, "locationID"=0, "interfaceID"=1} ("Source Info"), "domainID"=w411, "sideID"=w410, "locationID"=w409, "interfaceID"=w414) -> (w415:T11)
        n175 = Bundle By Name(cluster=T10 {"domainID"=0, "sideID"=0, "locationID"=0, "partitionID"=1} ("Source Info"), "domainID"=w411, "sideID"=w410, "locationID"=w409, "partitionID"=w408) -> (w412:T10)
        n176 = call "Format MAC into String.vi"("MAC"=w401) -> ("MAC String"=→"Destination MAC":string)  [unwired: 10 in]
        n177 = call <instrlib>:"Create ARINC-664 MAC (Source).vi"("Source Info"=w415) -> ("MAC-src"=w403:u8[])  [unwired: 9 in, 1 out]
        n178 = call <instrlib>:"Create ARINC-664 IP (Source).vi"("Source Info"=w412) -> ("ip address"=→"Source IP":string)  [unwired: 9 in, 1 out]
        n179 = for {
          tunnel: w403 -> [w436] mode=indexing
          shift-right: [w432] -> w399
          shift-left: "" -> [w431]
          n180 = Number To Hexadecimal String(1:i16 2 ("width (-)"), 2:w436) -> (0:w434:string)
          n181 = Concatenate Strings(w431, w434, ":" ("string")) -> (w432:string)
        }
        n182 = String Length(string=w399) -> (length=w398:i32)
        n183 = Merge Errors(w419) -> (w423:errorcluster)
        n184 = Decrement(x=w398) -> (x-1=w397:i32)
        n185 = String Subset(string=w399, length (rest)=w397) -> (substring=→"Source MAC":string)  [unwired: 1 in]
      }
      frame "Error" {
        # "#CodeRecommended - If you ever change the name of this \"Error\" message, you'll need to update the name in the Check Loop Error.vi as well."
        # "#CodeRecommended - Consider creating a system for logging errors in some way. These errors are for notification purposes only. Handling of specific errors should be performed in the message frames that generated the error."
        # "Error - Display an error dialog. This message is sent by the \"Error Handler\" VIs at the end of other loops in this application."
        n186 = Variant To Data(error in=w444, type=errorcluster {"status"=FALSE, "code"=0, "source"=""} ("error constant"), Variant=w442) -> (data=w440:errorcluster, error out=w437:errorcluster)
        n187 = call <vilib>:"Simple Error Handler.vi"("error in (no error)"=w440) -> ()  [unwired: 4 in, 5 out]
        n188 = Merge Errors(w437) -> (w439:errorcluster)
      }
      frame "Confirm Quit" {
        # "#CodeNeeded - If you want to provide an \"Are you sure\" dialog (or some other notification) before the application exits, place that code here. This message is typically sent from a Panel Close? event."
        # "Confirm Quit - Message that can confirm whether or not the user wants to exit the application."
        n189 = call-poly "Enqueue Message.vi"("Priority Message? (F)"=TRUE, "error in (no error)"=w452, "Message"="Cancel", "Message Queue"=w448) -> ("error out"=w449:errorcluster)  [unwired: 6 in, 1 out]
        n190 = Merge Errors(w449) -> (w450:errorcluster)
      }
      frame "---Copy This Frame---" {
        # "Duplicate this frame when creating new messages.  Change this comment in the duplicated frame to describe this message."
        n191 = Merge Errors(w456) -> (w454:errorcluster)
      }
      frame "Payload" {
        # "Duplicate this frame when creating new messages.  Change this comment in the duplicated frame to describe this message."
        n192 = local read "option"() -> (w463:u32)
        n193 = case shown="8" w463 {
          tunnel: w465 -> [_ w473 w478 w482 w487]
          tunnel: w464 -> [_ w472 w477 w483 w486]
          tunnel: [_ w469 w474 w479 w485] -> w457
          frame Default {
          }
          frame 1 {
            n194 = call-poly <instrlib>:"Create Payload.vi"("Bit Length"=w472, "Value"=u64 0, "Length"=w473) -> ("error out"=w469:errorcluster, "Payload (U8)"=w471:u8[])  [unwired: 6 in, 1 out]
            n195 = local write "Payload"(w471) -> ()
          }
          frame 2 {
            n196 = call-poly <instrlib>:"Create Payload.vi"("Bit Length"=w477, "Value"="Fill Value", "Length"=w478) -> ("error out"=w474:errorcluster, "Payload (U8)"=w476:u8[])  [unwired: 6 in, 1 out]
            n197 = local write "Payload"(w476) -> ()
          }
          frame 4 {
            n198 = call-poly <instrlib>:"Create Payload.vi"("Bit Length"=w483, "Interval"="Increment", "Start Value"="Start", "Length"=w482) -> ("error out"=w479:errorcluster, "Payload (U8)"=w484:u8[])  [unwired: 5 in, 1 out]
            n199 = local write "Payload"(w484) -> ()
          }
          frame 8 {
            n200 = call-poly <instrlib>:"Create Payload.vi"("Bit Length"=w486, "Length"=w487) -> ("error out"=w485:errorcluster, "Payload (U8)"=w488:u8[])  [unwired: 7 in, 1 out]
            n201 = local write "Payload"(w488) -> ()
          }
        }
        n202 = call <vilib>:"Clear Errors.vi"("error in (no error)"=w457) -> ()  [unwired: 5 in, 2 out]
        n203 = call-poly "Enqueue Message.vi"("error in (no error)"=w462, "Message Data"="Created payload" ("Message"), "Message"="Update Display", "Message Queue"=w459) -> ("error out"=w461:errorcluster)  [unwired: 6 in, 1 out]
        n204 = Merge Errors(w461) -> (w467:errorcluster)
      }
      frame "Exit" {
        # "Stop the VI"
        # "Release the message queue reference"
        # "#CodeNeeded - Add any required cleanup code here. Note that if 'Exit' was called as a result of an error, an error dialog will be displayed. Add any custom error handling for an 'Exit' condition here as well."
        # "Exit - Exit the application."
        n205 = Variant To Data(type=errorcluster {"status"=FALSE, "code"=0, "source"=""} ("error constant"), Variant=w490) -> (data=w491:errorcluster)  [unwired: 1 in, 1 out]
        n206 = call <vilib>:"Simple Error Handler.vi"("error in (no error)"=w491) -> ()  [unwired: 4 in, 5 out]
        n207 = call "Fire User Event - Stop.vi"("User Event - Stop"=w495) -> ("error out"=w494:errorcluster)  [unwired: 10 in]
        n208 = Release Queue(queue=w500, error in (no error)=w493) -> (error out=w497:errorcluster)  [unwired: 1 in, 2 out]
        n209 = Merge Errors(w494, w497) -> (w496:errorcluster)
        "Output Map" <- w489
      }
      frame "Cancel" {
        # "Stop the VI"
        # "Release the message queue reference"
        # "#CodeNeeded - Add any required cleanup code here. Note that if 'Exit' was called as a result of an error, an error dialog will be displayed. Add any custom error handling for an 'Exit' condition here as well."
        # "Exit - Exit the application."
        n210 = Variant To Data(type=errorcluster {"status"=FALSE, "code"=0, "source"=""} ("error constant"), Variant=w503) -> (data=w504:errorcluster)  [unwired: 1 in, 1 out]
        n211 = call <vilib>:"Simple Error Handler.vi"("error in (no error)"=w504) -> ()  [unwired: 4 in, 5 out]
        n212 = call "Fire User Event - Stop.vi"("User Event - Stop"=w508) -> ("error out"=w507:errorcluster)  [unwired: 10 in]
        n213 = Release Queue(queue=w513, error in (no error)=w506) -> (error out=w510:errorcluster)  [unwired: 1 in, 2 out]
        n214 = Merge Errors(w507, w510) -> (w509:errorcluster)
        "Cancelled" <- TRUE ("Cancelled")
      }
      frame Default {
        # "'Default' case only runs if there is a message that isn't defined in any of the other cases.  Output a programming error."
        n215 = xnode "Error Ring"("parameter 0"=w515) -> ("error out"=w516:errorcluster)
      }
    }
    n216 = call "Error Handler - Message Handling Loop.vi"("error in (no error)"=w43, "Message Queue"=w45) -> ("dup error in"=w44:errorcluster)  [unwired: 8 in, 1 out]
  }
  n217 = while {
    tunnel: w5 -> [w531]
    shift-right: [w529] -> w14
    shift-left: w10 -> [w530]
    tunnel: [w525] -> w11
    stop <- w527 stop-if-true
    # "Event Handling Loop"
    n218 = event shown="[5] \"Type of Frame\": Value Change" {
      selector: w530 -> [_ _ _ _ _ _ _ _ _ _ _ _ _ _]
      dyn-events: [_ _ _ _ _ _ _ _ _ _ _ _ _ _] -> w529
      timeout: _ -> [_ _ _ _ _ _ _ _ _ _ _ _ _ _]
      tunnel: [_ _ _ _ _ _ _ _ _ _ _ _ _ TRUE ("Discard?")] -> w527
      tunnel: w531 -> [w535 w539 w549 w553 w557 w561 w565 w588 w592 w597 w599 w604 w621 w624]
      tunnel: [w532 w536 w546 w550 _ _ w571 _ _ w596 _ w603 w620 _] -> w528
      tunnel: [w534 w538 w548 w552 w556 w560 w570 w587 w591 w595 w599 w602 w619 w624] -> w526
      event "Add / Update": Value Change {
        n219 = event-data() -> ()  [unwired: 1 in, 1 out]
        n220 = call-poly "Enqueue Message.vi"("Message"="Update", "Message Queue"=w535) -> ("error out"=w532:errorcluster, "dup Message Queue"=w534:refnum<queue>)  [unwired: 8 in]
      }
      event "Remove": Value Change {
        # "#CodeNeeded - Send the appropriate message for this user interface event."
        n221 = event-data() -> ()  [unwired: 1 in, 1 out]
        n222 = call-poly "Enqueue Message.vi"("Message"="Remove", "Message Queue"=w539) -> ("error out"=w536:errorcluster, "dup Message Queue"=w538:refnum<queue>)  [unwired: 8 in]
      }
      event "Clear Payload", "Fill Payload", "Increment Payload", "Random Payload", "Fill Value": Value Change {
        n223 = event-data() -> ()  [unwired: 1 in, 1 out]
        n224 = Build Array("Clear Payload", "Fill Payload", "Increment Payload", "Random Payload") -> (w541:bool[])
        n225 = call-poly "Enqueue Message.vi"("Message"="Payload", "Message Queue"=w549) -> ("error out"=w546:errorcluster, "dup Message Queue"=w548:refnum<queue>)  [unwired: 8 in]
        n226 = Boolean Array To Number(Boolean array=w541) -> (number=→"option":u32)
      }
      event "Payloads": Value Change {
        n227 = event-data() -> ()  [unwired: 1 in, 1 out]
        n228 = call-poly "Enqueue Message.vi"("Message"="ViewFrameInfo", "Message Queue"=w553) -> ("error out"=w550:errorcluster, "dup Message Queue"=w552:refnum<queue>)  [unwired: 8 in]
      }
      event "Location ID", "Interface ID", "Partition ID", "Domain ID", "Side ID", "Payload": Value Change {
        n229 = event-data() -> ()  [unwired: 1 in, 1 out]
        n230 = call-poly "Enqueue Message.vi"("Message Data"="Update" ("Message"), "Message"="Update Display", "Message Queue"=w557) -> ("dup Message Queue"=w556:refnum<queue>)  [unwired: 7 in, 1 out]
      }
      event Value Change {
        n231 = event-data() -> ()  [unwired: 1 in, 1 out]
        n232 = call-poly "Enqueue Message.vi"("Message Data"="Update" ("Message"), "Message"="Update Display", "Message Queue"=w561) -> ("dup Message Queue"=w560:refnum<queue>)  [unwired: 7 in, 1 out]
      }
      event "Payload Size": Value Change {
        n233 = event-data() -> ("OldVal"=w568:u32, "NewVal"=w566:u32)  [unwired: 1 in]
        n234 = Greater?(x=w568, y=w566) -> (0:w567:bool)
        n235 = local read "Payload"() -> (w572:u8[])
        n236 = case shown="False" w567 {
          tunnel: w572 -> [w577 w584]
          tunnel: [w578 w583] -> w569
          tunnel: w566 -> [w580 w582]
          tunnel: w565 -> [w575 w581]
          tunnel: [w575 w581] -> w564
          frame False {
            n237 = Initialize Array(u8 0 ("new element/subarray"), w580) -> (w576:u8[])
            n238 = Replace Array Subset(array=w576, new element=w577) -> (w578:u8[])  [unwired: 1 in]
          }
          frame True {
            n239 = Array Subset(array=w584, length=w582) -> (w583:u8[])  [unwired: 1 in]
          }
        }
        n240 = flat-sequence {
          tunnel: ["Update Display" ("Message")] -> w563
          tunnel: w569 -> [w573]
          frame #0 {
            n241 = local write "Payload"(w573) -> ()
          }
        }
        n242 = call-poly "Enqueue Message.vi"("Message Data"="Changed payload size." ("Message"), "Message"=w563, "Message Queue"=w564) -> ("error out"=w571:errorcluster, "dup Message Queue"=w570:refnum<queue>)  [unwired: 7 in]
      }
      event "Load": Value Change {
        n243 = event-data() -> ()  [unwired: 1 in, 1 out]
        n244 = call-poly "Enqueue Message.vi"("Message Data"="Load", "Message"="Load", "Message Queue"=w588) -> ("dup Message Queue"=w587:refnum<queue>)  [unwired: 7 in, 1 out]
      }
      event "Save": Value Change {
        n245 = event-data() -> ()  [unwired: 1 in, 1 out]
        n246 = call-poly "Enqueue Message.vi"("Message Data"=TRUE, "Message"="Save", "Message Queue"=w592) -> ("dup Message Queue"=w591:refnum<queue>)  [unwired: 7 in, 1 out]
      }
      event Panel Close? {
        # "Send the 'Confirm Quit' message if the user closes the panel of the VI. Discard the event so the 'Confirm Quit' message has a chance to run."
        n247 = event-data() -> ()  [unwired: 1 in, 1 out]
        n248 = call-poly "Enqueue Message.vi"("Priority Message? (F)"=TRUE, "Message"="Confirm Quit", "Message Queue"=w597) -> ("error out"=w596:errorcluster, "dup Message Queue"=w595:refnum<queue>)  [unwired: 7 in]
        n249 = event-data("Discard?"=TRUE) -> ()  [unwired: 1 in, 1 out]
      }
      event Application Instance Close {
        # "#CodeRecommended - When a project closes, all VIs within that project are aborted and leave memory. However, any code placed in this event frame is guaranteed to run to completion, so add any cleanup code that absolutely must happen here."
        n250 = event-data() -> ()  [unwired: 1 in, 1 out]
      }
      event "Exit": Value Change {
        n251 = event-data() -> ()  [unwired: 1 in, 1 out]
        n252 = call "prompt - save and close.vi"() -> ("message"=w600:string)  [unwired: 11 in]
        n253 = Two Button Dialog(message=w600) -> (T button?=w601:bool)  [unwired: 2 in]
        n254 = case shown="False" w601 {
          tunnel: w604 -> [w605 w610]
          tunnel: [_ w609] -> w603
          tunnel: [w605 w608] -> w602
          frame False {
          }
          frame True {
            n255 = for {
              tunnel: [w615] -> w609
              shift-right: [w614] -> w608
              shift-left: w610 -> [w616]
              tunnel: string[] ["Save", "Exit"] ("Message") -> [w613] mode=indexing
              tunnel: TRUE ("Priority Message? (F)") -> [w612]
              n256 = call-poly "Enqueue Message.vi"("Priority Message? (F)"=w612, "Message Data"=FALSE ("Priority Message? (F)"), "Message"=w613, "Message Queue"=w616) -> ("error out"=w615:errorcluster, "dup Message Queue"=w614:refnum<queue>)  [unwired: 6 in]
            }
          }
        }
      }
      event "Cancel": Value Change {
        n257 = event-data() -> ()  [unwired: 1 in, 1 out]
        n258 = call-poly "Enqueue Message.vi"("Priority Message? (F)"=TRUE, "Message"="Cancel", "Message Queue"=w621) -> ("error out"=w620:errorcluster, "dup Message Queue"=w619:refnum<queue>)  [unwired: 7 in]
      }
      event User Event {
        # "The Message Handling Loop processed an \"Exit\" message, which fired this event to stop the Event Handling Loop."
        n259 = event-data() -> ()  [unwired: 1 in, 1 out]
        n260 = local write "Display Message"("\"Exit\" button pressed" ("VI Stopped")) -> ()
      }
    }
    n261 = call "Error Handler - Event Handling Loop.vi"("error in (no error)"=w528, "Message Queue"=w526) -> ("dup error in"=w525:errorcluster)  [unwired: 8 in, 1 out]
  }
  n262 = disable-structure shown="Disabled" {
    frame Disabled {
      (unwired) "Update" ("text")
      n263 = Unbundle By Name() -> ("Add"=w625:refnum<vi>)  [unwired: 1 in]
      n264 = call "Set Boolean Button Text.vi"("boolean ref in"=w625) -> ()  [unwired: 10 in, 1 out]
    }
    frame Enabled {
    }
  }
  n265 = Unregister For Events(event registration refnum=w14, error in=w11) -> (error out=w15:errorcluster)
  n266 = Merge Errors(w15, w18) -> (w16:errorcluster)
  n267 = call "Destroy User Event - Stop.vi"("error in (no error)"=w16, "User Event - Stop"=w9) -> ("error out"=w12:errorcluster)  [unwired: 9 in]
  n268 = disable-structure shown="Default" {
    disable-tunnel: w12 -> [w626 _]
    frame condition #0 (active) {
      "error out" <- w626
    }
    frame condition #1 {
      # "Call Quit LabVIEW if running as a built application."
      n269 = Quit LabVIEW() -> ()  [unwired: 1 in]
    }
  }
